vi "Function.vi"(8 "error in (no error)":errorcluster, 10 "Numeric":T1, 11 "Two Terminal in":refnum<class "AbsComp_One Term_U32.lvclass">) -> (0 "error out":errorcluster, 2 "Result":bool, 3 "Two Terminal out":refnum<class "AbsComp_One Term_U32.lvclass">)   [LabVIEW 2021, in "AbsComp_One Term_U32.lvclass"]
uses:
  AbsComp_One Term_U32.lvclass
  Support/Data Type.ctl
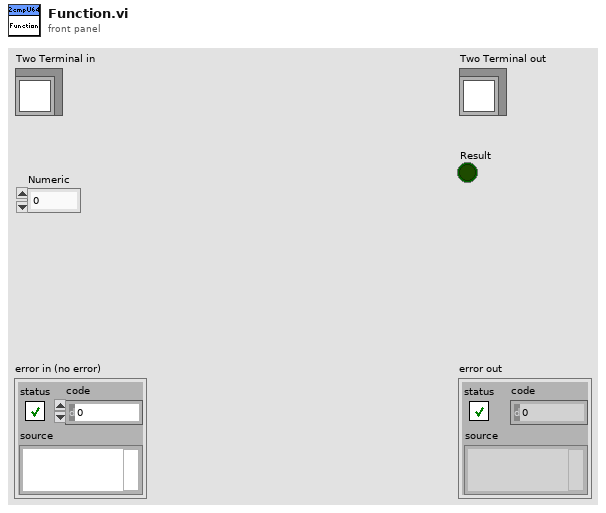
[diagram p1: front panel]
types:
  T1 = typedef "AbsComp_One Term_U32.lvclass/Data Type.ctl" = u32
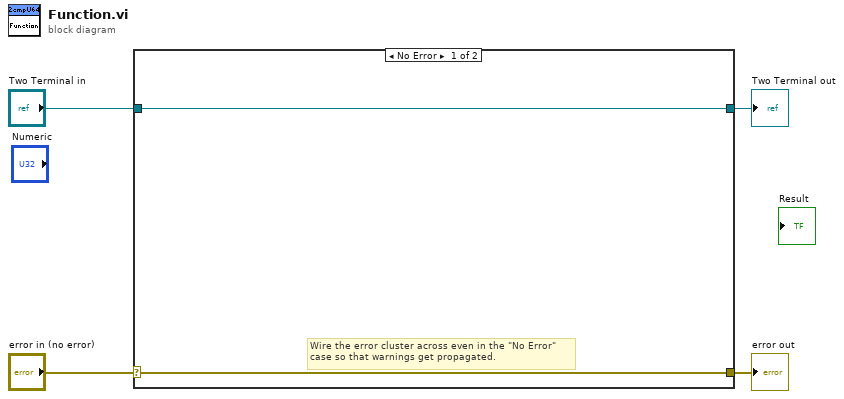
[diagram p0: block diagram]
diagram:
  n1 = case shown="No Error" "error in (no error)" {
    selector: "error in (no error)" -> [w5 w8]
    tunnel: [w5 w8] -> w3
    tunnel: [w6 w7] -> w1
    tunnel: "Two Terminal in" -> [w6 w7]
    frame No Error {
      # "Wire the error cluster across even in the \"No Error\"\ncase so that warnings get propagated."
    }
    frame Error {
    }
  }
  "error out" <- w3
  "Two Terminal out" <- w1
